vi "Add Selected Ctrl Properties.vi"(1 "Data Cluster In":T1) -> (0 "Data Cluster out":T1)   [LabVIEW 2020, in "Control Property Tree.lvlib"]
uses:
  Control Property Tree.lvlib
  Module Data--cluster.ctl
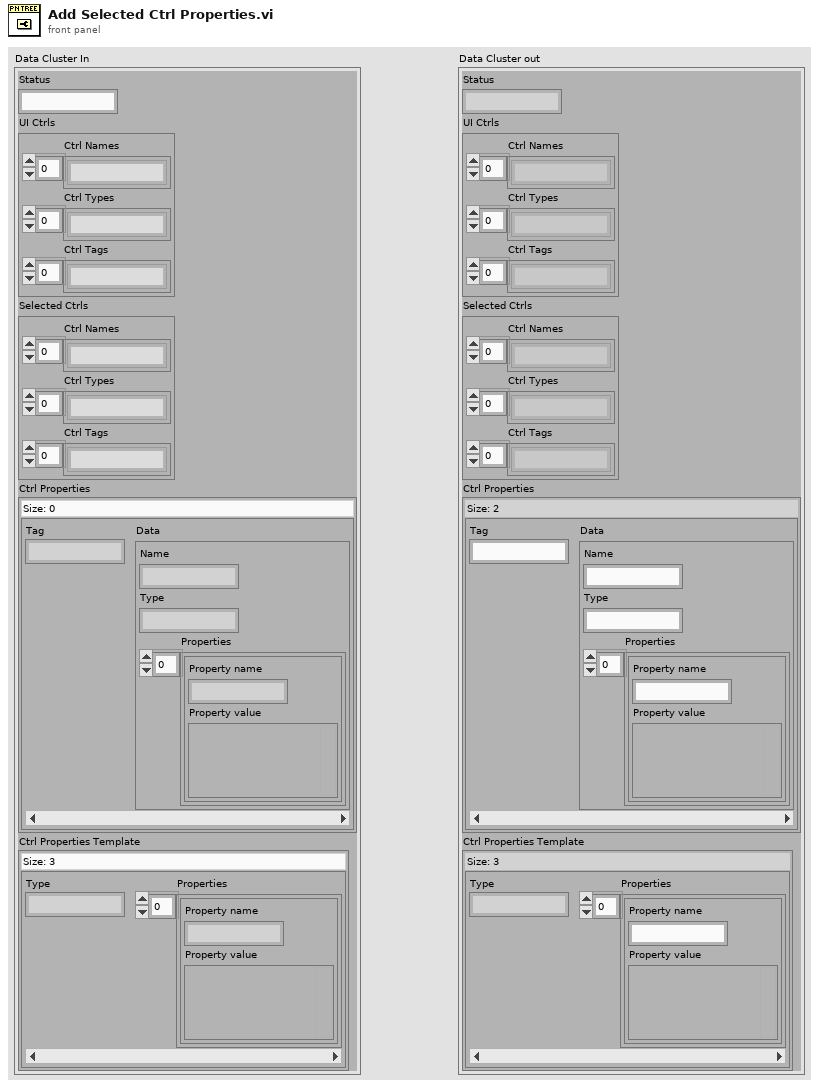
[diagram p1: front panel]
types:
  T1 = typedef "Control Property Tree.lvlib/Module Data--cluster.ctl" = cluster{"Status":string, "UI Ctrls":cluster{"Ctrl Names":string[], "Ctrl Types":string[], "Ctrl Tags":string[]}, "Selected Ctrls":cluster{"Ctrl Names":string[], "Ctrl Types":string[], "Ctrl Tags":string[]}, "Ctrl Properties":map{string, cluster{"Name":string, "Type":string, "Properties":cluster{"Property name":string, "Property value":variant}[]}}, "Ctrl Properties Template":map{string, cluster{"Property name":string, "Property value":variant}[]}}
  T2 = map{string, cluster{"Name":string, "Type":string, "Properties":cluster{"Property name":string, "Property value":variant}[]}}
  T3 = map{string, cluster{"Property name":string, "Property value":variant}[]}
  T4 = cluster{"Name":string, "Type":string, "Properties":cluster{"Property name":string, "Property value":variant}[]}
  T5 = cluster{"Property name":string, "Property value":variant}[]
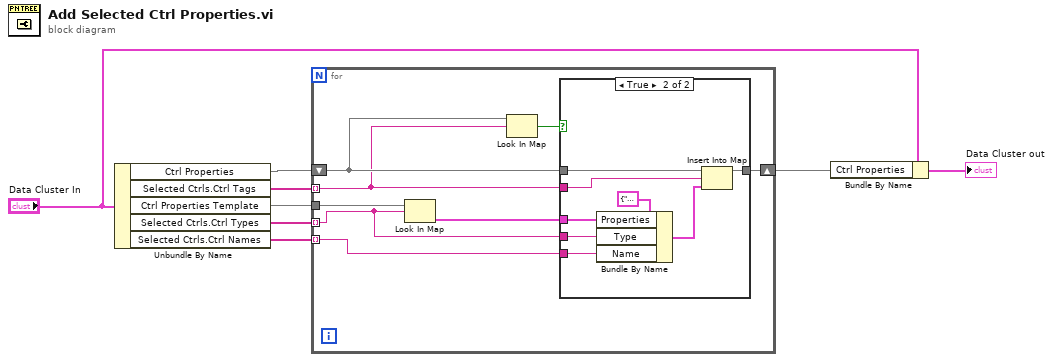
[diagram p0: block diagram]
diagram:
  n1 = Unbundle By Name("Data Cluster In") -> ("Ctrl Properties"=w5:T2, "Selected Ctrls.Ctrl Tags"=w4:string[], "Ctrl Properties Template"=w6:T3, "Selected Ctrls.Ctrl Types"=w8:string[], "Selected Ctrls.Ctrl Names"=w7:string[])
  n2 = for {
    tunnel: w8 -> [w14] mode=indexing
    tunnel: w7 -> [w13] mode=indexing
    tunnel: w6 -> [w16]
    tunnel: w4 -> [w9] mode=indexing
    shift-right: [w12] -> w2
    shift-left: w5 -> [w10]
    n3 = Look In Map(map=w16, key=w14) -> (value=w15:T5)  [unwired: 1 in, 1 out]
    n4 = Look In Map(map=w10, key=w9) -> (key not found?=w11:bool)  [unwired: 1 in, 1 out]
    n5 = case shown="True" w11 {
      tunnel: w10 -> [w17 w25]
      tunnel: w9 -> [_ w24]
      tunnel: w15 -> [_ w22]
      tunnel: w14 -> [_ w21]
      tunnel: w13 -> [_ w20]
      tunnel: [w17 w18] -> w12
      frame False {
      }
      frame True {
        n6 = Bundle By Name(cluster=T4 {"Name"="", "Type"="", "Properties"=[]} ("value"), "Properties"=w22, "Type"=w21, "Name"=w20) -> (w19:T4)
        n7 = Insert Into Map(map in=w25, key=w24, value=w19) -> (map out=w18:T2)  [unwired: 2 out]
      }
    }
  }
  n8 = Bundle By Name(cluster="Data Cluster In", "Ctrl Properties"=w2) -> (→"Data Cluster out":T1)
